vi "BundleParameters.vi"(8 "Wsp. szczytu":dbl, 9 "RMS":dbl, 10 "Kurtoza":dbl, 11 "Parameters labels":T1[](array[typedef])) -> (3 "Parameters":dbl[](array[numeric]))   [LabVIEW 2019]
uses:
  MobileAnalyzer/mainVIs/analyzeAccelerationDataVIs/calculateFaultIndicatorsVIs/FaultParameter.ctl
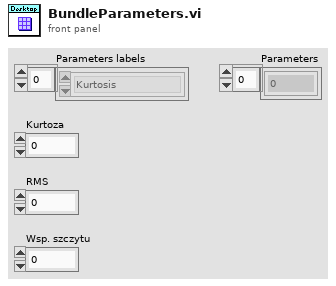
[diagram p1: front panel]
types:
  T1 = typedef "FaultParameter.ctl" = enum16{"Kurtosis", "RMS", "Crest factor"}
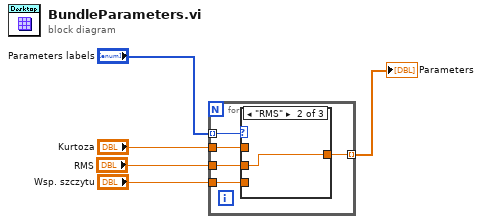
[diagram p0: block diagram]
diagram:
  n1 = for {
    tunnel: "Parameters labels" -> [w10] mode=indexing
    tunnel: [w9] -> w1 mode=indexing
    tunnel: "Kurtoza" -> [w8]
    tunnel: "RMS" -> [w7]
    tunnel: "Wsp. szczytu" -> [w6]
    n2 = case shown="\"RMS\"" w10 {
      tunnel: [w11 w12 w13] -> w9
      tunnel: w8 -> [w11 _ _]
      tunnel: w7 -> [_ w12 _]
      tunnel: w6 -> [_ _ w13]
      frame "Kurtosis" {
      }
      frame "RMS" {
      }
      frame "Crest factor" {
      }
    }
  }
  "Parameters" <- w1
